vi "RT_Parse Data.vi"(11 "Data In":u8[](array[numeric]) format="%.0x") -> (3 "Data Out":T1)   [LabVIEW 2018]
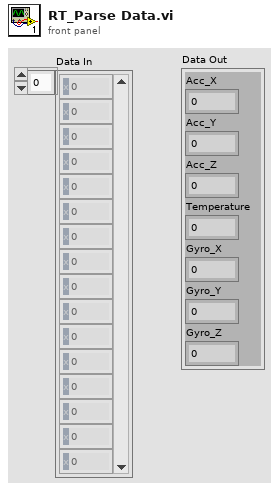
[diagram p1: front panel]
types:
  T1 = cluster{"Acc_X":dbl, "Acc_Y":dbl, "Acc_Z":dbl, "Temperature":dbl, "Gyro_X":dbl, "Gyro_Y":dbl, "Gyro_Z":dbl}
  T2 = cluster{"[0]":u16, "[1]":u16, "[2]":u16, "[3]":u16, "[4]":u16, "[5]":u16, "[6]":u16}
  T3 = cluster{"[0]":i16, "[1]":i16, "[2]":i16, "[3]":i16, "[4]":i16, "[5]":i16, "[6]":i16}
  T4 = cluster{"[0]":dbl, "[1]":dbl, "[2]":dbl, "[3]":dbl, "[4]":dbl, "[5]":dbl, "[6]":dbl}
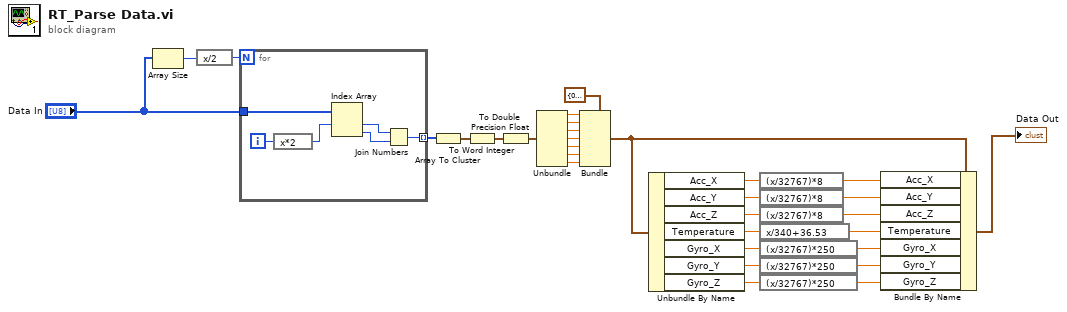
[diagram p0: block diagram]
diagram:
  n1 = Array Size(array="Data In") -> (size(s)=w30:i32)
  n2 = expression code="x/2"(w30) -> (w29:i32)
  n3 = for {
    N: w29 -> [_]
    tunnel: "Data In" -> [w37]
    tunnel: [w32] -> w28 mode=indexing
    i -> [w36]
    n4 = expression code="x*2"(w36) -> (w35:i32)
    n5 = Index Array(array=w37, index #1=w35) -> (element #1=w33:u8, element #2=w34:u8)  [unwired: 1 in]
    n6 = Join Numbers(hi=w33, lo=w34) -> ((hi.lo)=w32:u16)
  }
  n7 = Array To Cluster(array=w28) -> (cluster=w9:T2)
  n8 = To Word Integer(number=w9) -> (16bit integer=w8:T3)
  n9 = To Double Precision Float(number=w8) -> (double precision float=w7:T4)
  n10 = Unbundle(w7) -> ("[0]"=w26:dbl, "[1]"=w25:dbl, "[2]"=w24:dbl, "[3]"=w23:dbl, "[4]"=w22:dbl, "[5]"=w21:dbl, "[6]"=w20:dbl)
  n11 = Bundle(cluster=T1 {"Acc_X"=0.0, "Acc_Y"=0.0, "Acc_Z"=0.0, "Temperature"=0.0, "Gyro_X"=0.0, "Gyro_Y"=0.0, "Gyro_Z"=0.0} ("Data Out"), "Acc_X"=w26, "Acc_Y"=w25, "Acc_Z"=w24, "Temperature"=w23, "Gyro_X"=w22, "Gyro_Y"=w21, "Gyro_Z"=w20) -> (w18:T1)
  n12 = Unbundle By Name(w18) -> ("Acc_X"=w15:dbl, "Acc_Y"=w13:dbl, "Acc_Z"=w12:dbl, "Temperature"=w19:dbl, "Gyro_X"=w6:dbl, "Gyro_Y"=w4:dbl, "Gyro_Z"=w3:dbl)
  n13 = expression code="(x/32767)*8"(w15) -> (w14:dbl)
  n14 = expression code="(x/32767)*8"(w13) -> (w11:dbl)
  n15 = expression code="(x/32767)*8"(w12) -> (w10:dbl)
  n16 = expression code="x/340+36.53"(w19) -> (w17:dbl)
  n17 = expression code="(x/32767)*250"(w6) -> (w5:dbl)
  n18 = expression code="(x/32767)*250"(w4) -> (w2:dbl)
  n19 = expression code="(x/32767)*250"(w3) -> (w1:dbl)
  n20 = Bundle By Name(cluster=w18, "Acc_X"=w14, "Acc_Y"=w11, "Acc_Z"=w10, "Temperature"=w17, "Gyro_X"=w5, "Gyro_Y"=w2, "Gyro_Z"=w1) -> (→"Data Out":T1)
